vi "TSVD.vi"(10 "b":T1 caption="b（待输入误差）", 11 "S表":dbl[][](array[numeric])) -> (2 "k值":i32, 3 "x_TSVD":T1 caption="x_TSVD B")   [LabVIEW 2017]
uses:
  <vilib>/Analysis/Matrix/Datatypes/RealMatrix.ctl
  <vilib>/Analysis/7linalg.llb/Real Transpose Matrix.vi
  <vilib>/Analysis/baseanly.llb/Real A x B.vi
  <vilib>/Analysis/7linalg.llb/Real SVD Decomposition.vi
  <vilib>/Analysis/Matrix/Numeric/Conversions/Array To Matrix - RA2.vi
  <vilib>/Analysis/NI_AALPro.lvlib
  <vilib>/Analysis/NI_AALBase.lvlib
  <vilib>/Analysis/Matrix/NI_Matrix.lvlib
panel:
  out "error":i32 caption="错误"
  out "Matrix Transpose":T1 caption="矩阵转置"
  out "数组":dbl[](array[numeric])
  out "temp2":T1 caption="temp2=temp1与1/x逐元素相乘"
  out "temp1":T1 caption="temp1(k*1)"
  out "1/x":dbl[][](array[numeric])
  out "Uk":dbl[][](array[numeric])
  out "Vk":T1 caption="矩阵V"
  out "Matrix S":T1 caption="矩阵S"
  out "Matrix U":T1 caption="矩阵U"
  out "Vector S":dbl[][](array[numeric]) caption="向量Sk"
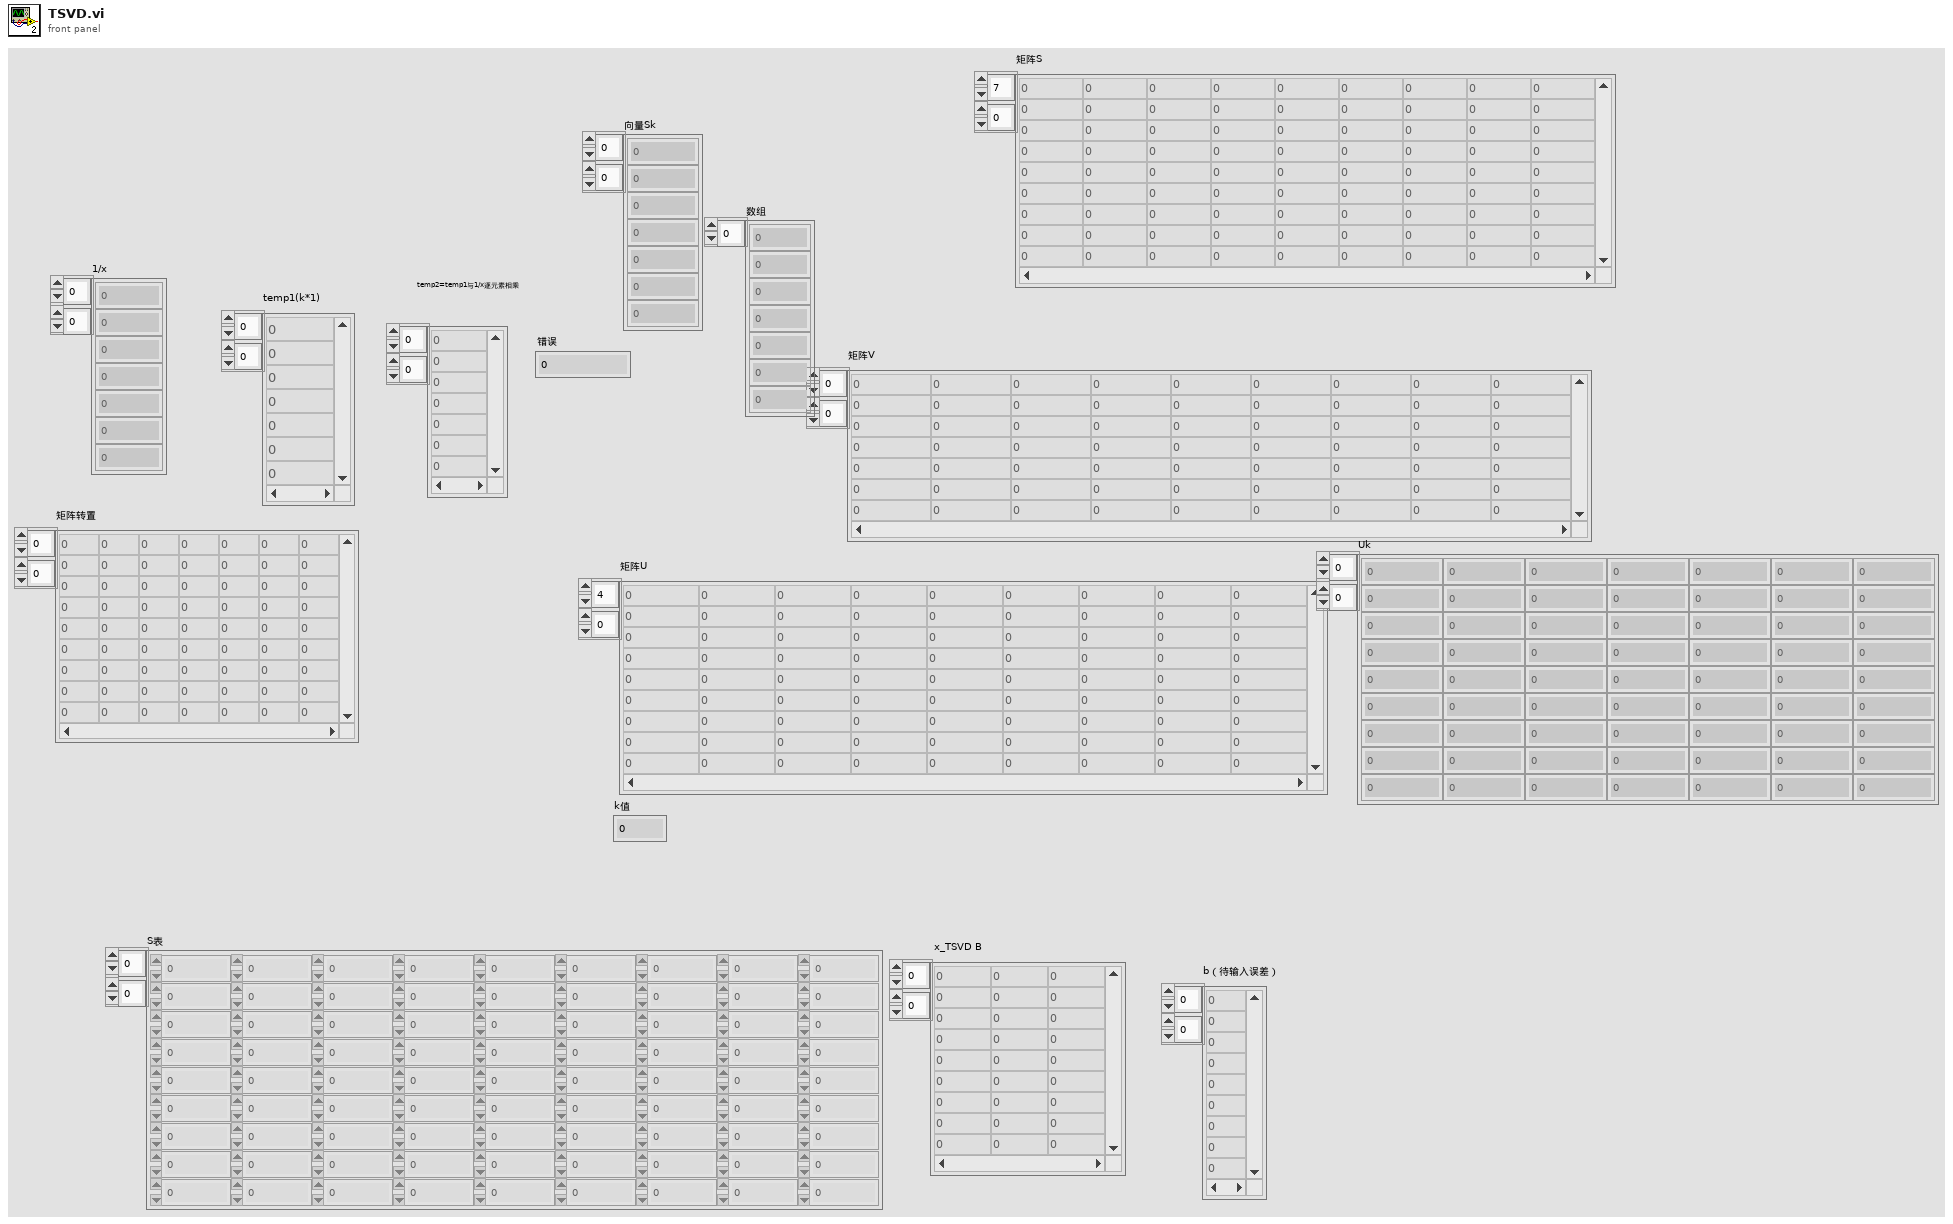
[diagram p1: front panel]
types:
  T1 = typedef "NI_Matrix.lvlib/RealMatrix.ctl" = dbl[][]
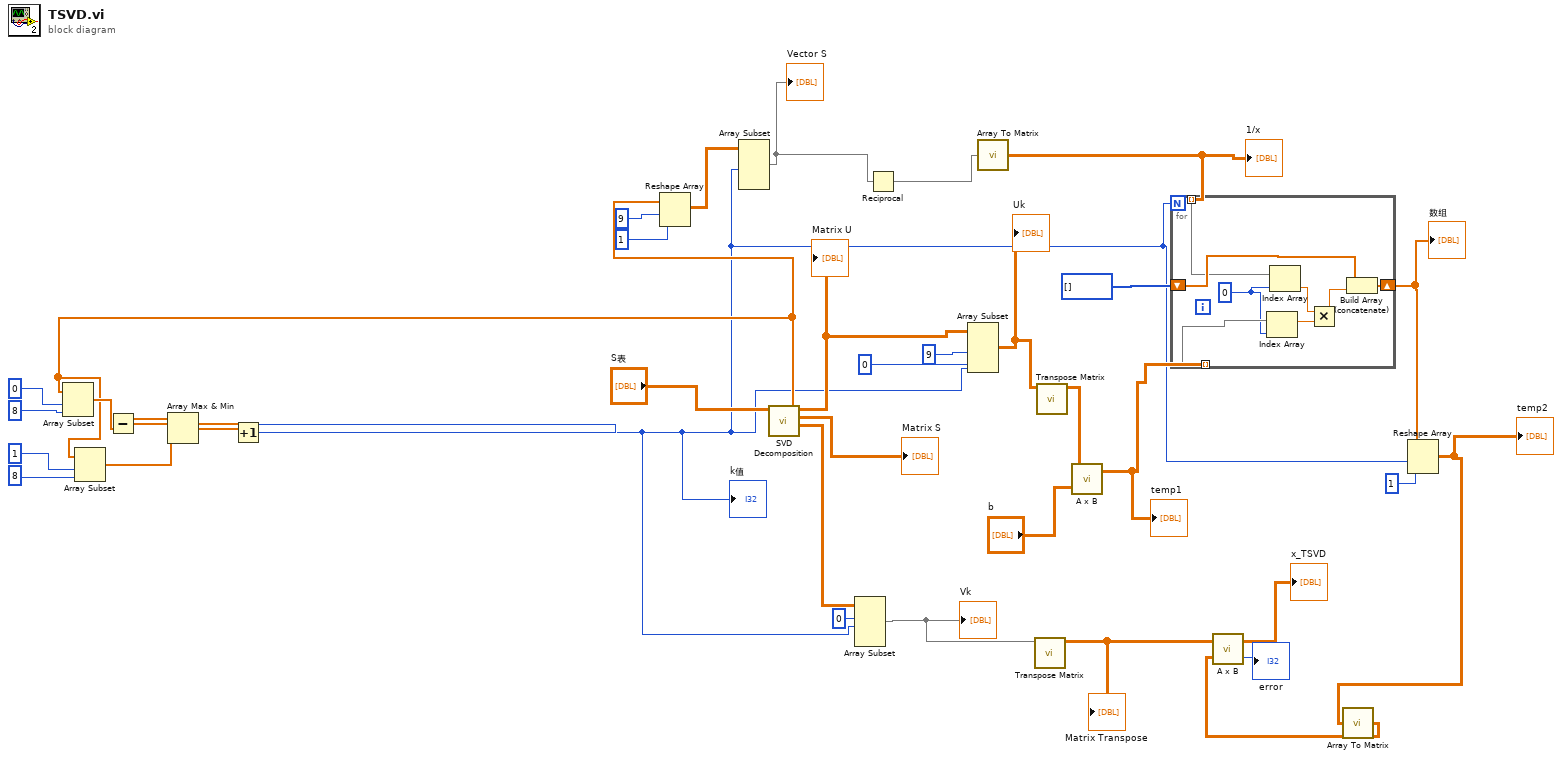
[diagram p0: block diagram]
diagram:
  n1 = call-poly <vilib>:"SVD Decomposition.vi"("A"="S表") -> ("Matrix V"=w15:T1, "Matrix S"=→"Matrix S":T1, "Matrix U"=w26:T1, "Vector S"=w20:dbl[])  [unwired: 6 in, 1 out]
  "Matrix U" <- w26
  n2 = Array Subset(array=w20, index=0 ("索引"), length=8 ("索引")) -> (w29:dbl[])
  n3 = Array Subset(array=w20, index=1 ("索引"), length=8 ("索引")) -> (w30:dbl[])
  n4 = Subtract(x=w30, y=w29) -> (x-y=w28:dbl[])
  n5 = Array Max & Min(array=w28) -> (max index (indices)=w27:i32)  [unwired: 3 out]
  n6 = Increment(x=w27) -> (x+1=w1:i32)
  "k值" <- w1
  n7 = Reshape Array(w20, 9 ("维数大小"), 1 ("维数大小")) -> (w17:dbl[][])
  n8 = Array Subset(array=w17, length (row)=w1) -> (w16:dbl[][])  [unwired: 3 in]
  "Vector S" <- w16
  n9 = Array Subset(array=w15, index (row)=0 ("索引"), length (row)=w1) -> (w12:T1)  [unwired: 2 in]
  "Vk" <- w12
  n10 = Reciprocal(x=w16) -> (1/x=w6:dbl[][])
  n11 = Array Subset(array=w26, length (row)=9 ("长度"), index (col)=0 ("索引"), length (col)=w1) -> (w23:T1)  [unwired: 1 in]
  "Uk" <- w23
  n12 = call-poly <vilib>:"Array To Matrix.vi"("Real 2D Array"=w6) -> ("Real Matrix"=w5:T1)
  "1/x" <- w5
  n13 = call-poly <vilib>:"Transpose Matrix.vi"("Input Matrix"=w12) -> ("Matrix Transpose"=w11:T1)  [unwired: 9 in, 1 out]
  "Matrix Transpose" <- w11
  n14 = call-poly <vilib>:"Transpose Matrix.vi"("Input Matrix"=w23) -> ("Matrix Transpose"=w22:T1)  [unwired: 9 in, 1 out]
  n15 = call-poly <vilib>:"A x B.vi"("B"="b", "A"=w22) -> ("A x B"=w9:T1)  [unwired: 1 out]
  "temp1" <- w9
  n16 = for {
    N: w1 -> [_]
    shift-right: [w41] -> w8
    shift-left: i32[] [] -> [w40]
    tunnel: w9 -> [w44] mode=indexing
    tunnel: w5 -> [w39] mode=indexing
    w37 = 0 ("索引")
    n17 = Index Array(array=w44, index=w37) -> (element=w43:dbl)
    n18 = Index Array(array=w39, index=w37) -> (element=w38:dbl)
    n19 = Multiply ("Multiply.vi")(x=w38, y=w43) -> (x*y=w42:dbl)
    n20 = Build Array (concatenate)(w40, w42) -> (w41:dbl[])
  }
  "数组" <- w8
  n21 = Reshape Array(w8, w1, 1 ("维数大小")) -> (w3:dbl[][])
  "temp2" <- w3
  n22 = call-poly <vilib>:"Array To Matrix.vi"("Real 2D Array"=w3) -> ("Real Matrix"=w2:T1)
  n23 = call-poly <vilib>:"A x B.vi"("B"=w2, "A"=w11) -> ("error"=→"error":i32, "A x B"=→"x_TSVD":T1)
